vi "Destroy.vi"(8 "error in (no error)":errorcluster, 11 "FastTreeView in":refnum<class "FastTreeView.lvclass">) -> (0 "error out":errorcluster, 3 "FastTreeView out":refnum<class "FastTreeView.lvclass">)   [LabVIEW 2025, in "FastTreeView.lvclass"]
uses:
  FastTreeView.lvclass
  FastTreeView.lvclass/FastTreeView.ctl
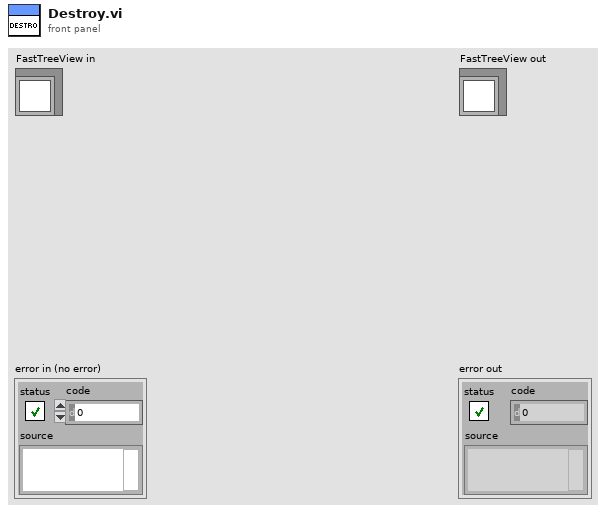
[diagram p1: front panel]
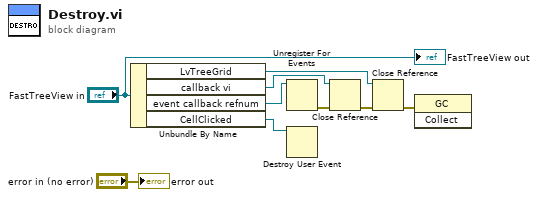
[diagram p0: block diagram]
diagram:
  n1 = Unbundle By Name("FastTreeView in") -> ("LvTreeGrid"=w7:refnum<k24>, "callback vi"=w2:refnum<vi>, "event callback refnum"=w6:refnum<k27>, "CellClicked"=w5:refnum<user-event>)
  n2 = Unregister For Events(event registration refnum=w6) -> (error out=w4:errorcluster)  [unwired: 1 in]
  n3 = Destroy User Event(user event=w5) -> ()  [unwired: 1 in, 1 out]
  n4 = Close Reference(reference=w2, error in (no error)=w4) -> (error out=w3:errorcluster)
  n5 = Close Reference(reference=w7, error in (no error)=w3) -> (error out=w1:errorcluster)
  n6 = invoke class="GC" method="Collect"(error in=w1) -> ()  [unwired: 2 in, 3 out]
  "error out" <- "error in (no error)"
  "FastTreeView out" <- "FastTreeView in"
